vi "fgv_error_rc.vi"(7 "cmd":T1, 11 "Error":T2) -> (3 "Error 2":T2)   [LabVIEW 2019]
uses:
  error_rc.ctl
  _ctrl/init-r-w.ctl
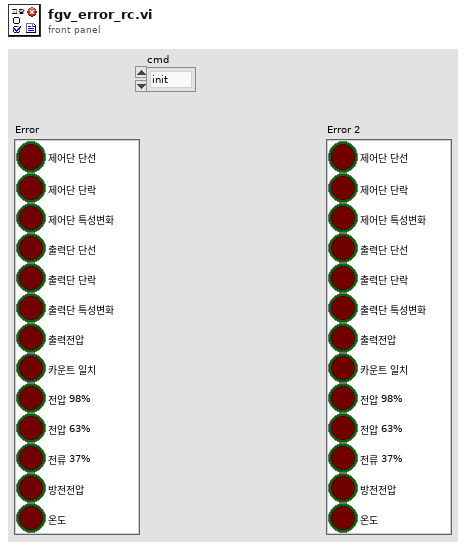
[diagram p1: front panel]
types:
  T1 = typedef "init-r-w.ctl" = enum16{"init", "read", "write"}
  T2 = typedef "error_rc.ctl" = cluster{"제어단 단선":bool, "제어단 단락":bool, "제어단 특성변화":bool, "출력단 단선":bool, "출력단 단락":bool, "출력단 특성변화":bool, "출력전압":bool, "카운트 일치":bool, "전압 98%":bool, "전압 63%":bool, "전류 37%":bool, "방전전압":bool, "온도":bool}
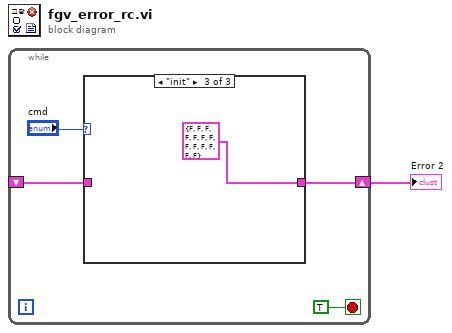
[diagram p0: block diagram]
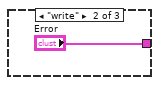
[diagram p3: hidden frame]
diagram:
  n1 = while {
    shift-right: [w4] -> w1
    shift-left: _ -> [w3]
    stop <- TRUE stop-if-true
    n2 = case shown="\"init\"" "cmd" {
      tunnel: [w6 "Error" T2 {"제어단 단선"=FALSE, "제어단 단락"=FALSE, "제어단 특성변화"=FALSE, "출력단 단선"=FALSE, "출력단 단락"=FALSE, "출력단 특성변화"=FALSE, "출력전압"=FALSE, "카운트 일치"=FALSE, "전압 98%"=FALSE, "전압 63%"=FALSE, "전류 37%"=FALSE, "방전전압"=FALSE, "온도"=FALSE} ("Error")] -> w4
      tunnel: w3 -> [w6 _ _]
      frame "read", Default {
      }
      frame "write" {
      }
      frame "init" {
      }
    }
  }
  "Error 2" <- w1
